vi "FlatToRichpumploop_Controls.vi"(5 "OutputClusterType":T1, 11 "InputCluster":T2) -> (3 "OutputCluster":T1)   [LabVIEW 2024, in "pumploop_client.lvlib"]
uses:
  pumploop_client.lvlib
  pumploop_Controls_Flat.ctl
  pumploop_Controls.ctl
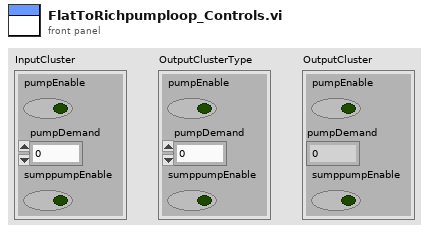
[diagram p1: front panel]
types:
  T1 = typedef "pumploop_client.lvlib/pumploop_Controls.ctl" = cluster{"pumpEnable":bool, "pumpDemand":sgl, "sumppumpEnable":bool}
  T2 = typedef "pumploop_client.lvlib/pumploop_Controls_Flat.ctl" = cluster{"pumpEnable":bool, "pumpDemand":sgl, "sumppumpEnable":bool}
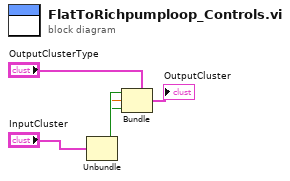
[diagram p0: block diagram]
diagram:
  n1 = Unbundle "Unbundle"("InputCluster") -> ("pumpEnable"=w3:bool, "pumpDemand"=w2:sgl, "sumppumpEnable"=w1:bool)
  n2 = Bundle "Bundle"(cluster="OutputClusterType", "pumpEnable"=w3, "pumpDemand"=w2, "sumppumpEnable"=w1) -> (→"OutputCluster":T1)
